vi "CCD_cinfig_to_INP.vi"(1 "Ask If Ok To Save":bool, 2 "Timing and Temperature":T4={"Exposure"=0.001, "Collection Mode"=1, "Timing Mode"=1, "Trigger Edge"=1, "Temperature"=-10.0} {"Temperature" format="%.2f"; "Trigger Edge" max=7 step=1; "Timing Mode" min=1 max=20 step=1; "Exposure" min=0.0 step=0.001 format="%.3f"}, 6 "Custom Chip":T1, 7 "ADC and Cleans":T3={"ADC Speed"=-2, "ADC Gain"=-1, "ADC Offset"=-1, "Readout Port"=-1, "Num Cleans"=1, "Num Strips per Clean"=10, "Mini Block Size"=2, "Num Min Blocks"=3, "Continous Cleans"=FALSE, "Skip Serial Reg Clean"=FALSE} {"Readout Port" min=-1 step=1; "ADC Offset" min=-1 step=1; "ADC Gain" min=-1 step=1; "ADC Speed" min=-3 step=1}, 8 "error in (no error)":errorcluster, 9 "Shutter and Logic Out":T2={"Shutter State"=2, "Open Comp Time "=0, "Close Comp Time"=0, "Logic Out Setting"=1, "Logic Out Invert"=FALSE} {"Logic Out Setting" min=1 max=14 step=1}, 10 "Camera Number":u32=1, 11 "Full File Path":string) -> (0 "error out":errorcluster)   [LabVIEW 2015]
uses:
  <vilib>/Utility/config.llb/Write Key (String).vi
  <vilib>/Utility/config.llb/Write Key (Double).vi
  <vilib>/Utility/config.llb/Write Key (U32).vi
  <vilib>/Utility/config.llb/Write Key (Boolean).vi
  <vilib>/Utility/config.llb/Write Key (I32).vi
  <vilib>/Utility/config.llb/NI_LVConfig.lvlib
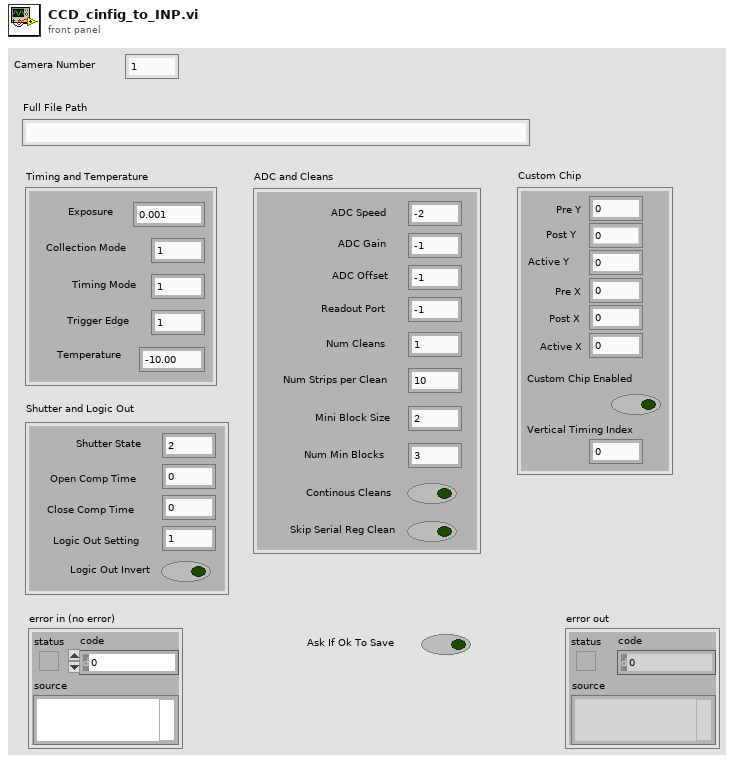
[diagram p1: front panel]
types:
  T1 = cluster{"Pre Y":u32, "Post Y":u32, "Active Y":u32, "Pre X":u32, "Post X":u32, "Active X":u32, "Custom Chip Enabled":bool, "Vertical Timing Index":u32}
  T2 = cluster{"Shutter State":u16, "Open Comp Time ":u32, "Close Comp Time":u32, "Logic Out Setting":u32, "Logic Out Invert":bool}
  T3 = cluster{"ADC Speed":i32, "ADC Gain":i32, "ADC Offset":i32, "Readout Port":i32, "Num Cleans":u32, "Num Strips per Clean":u32, "Mini Block Size":u32, "Num Min Blocks":u32, "Continous Cleans":bool, "Skip Serial Reg Clean":bool}
  T4 = cluster{"Exposure":dbl, "Collection Mode":u32, "Timing Mode":u32, "Trigger Edge":u32, "Temperature":dbl}
  T5 = typedef "NI_LVConfig.lvlib/Config Data RefNum.ctl" = refnum<k1>
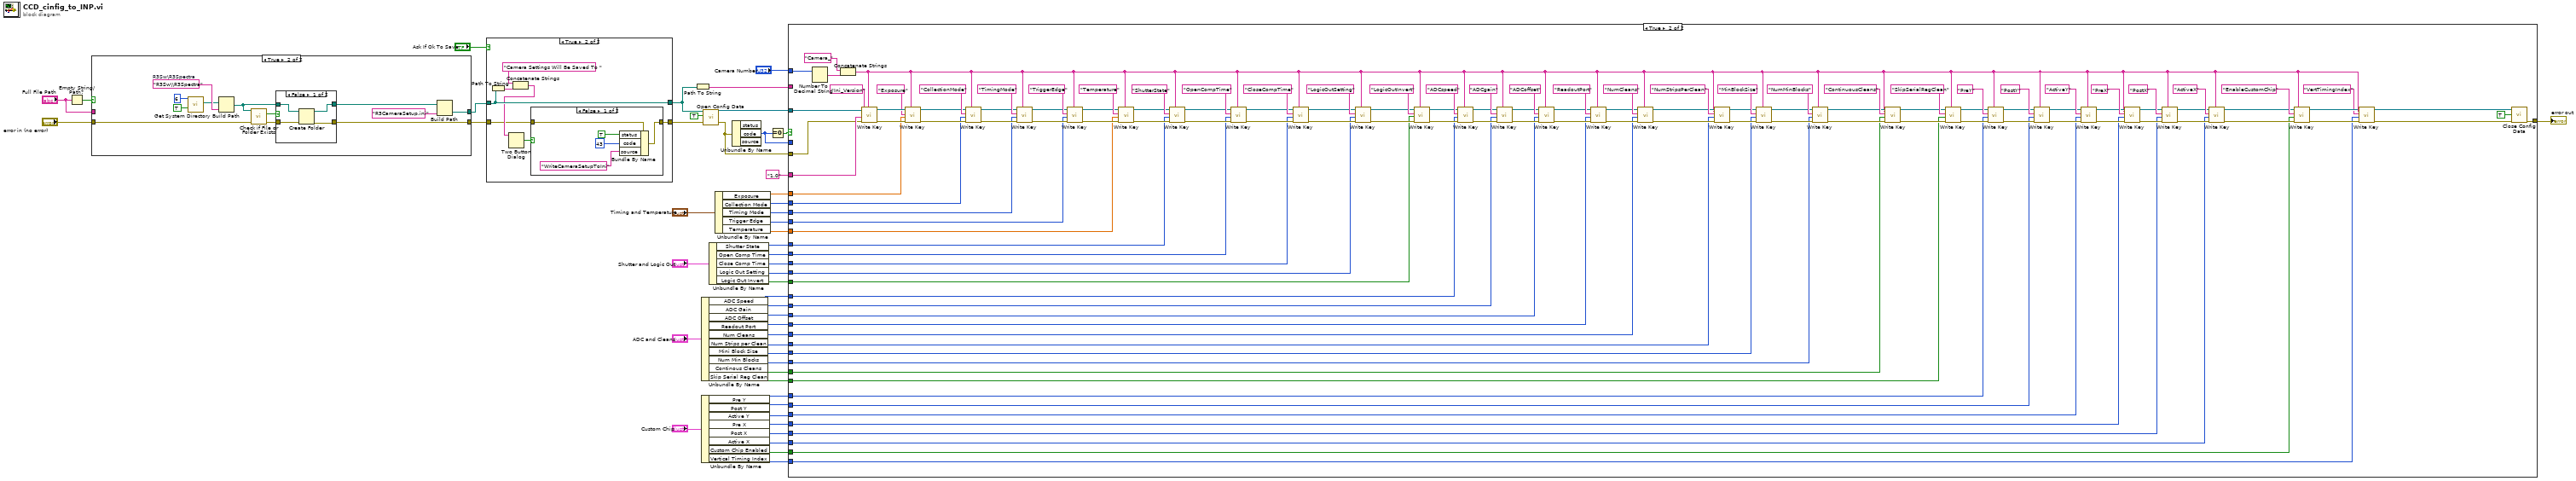
[diagram p0: block diagram]
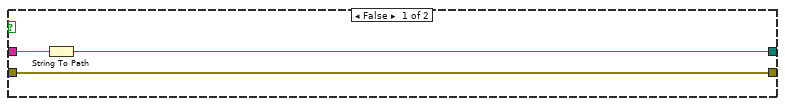
[diagram p4: hidden frame]
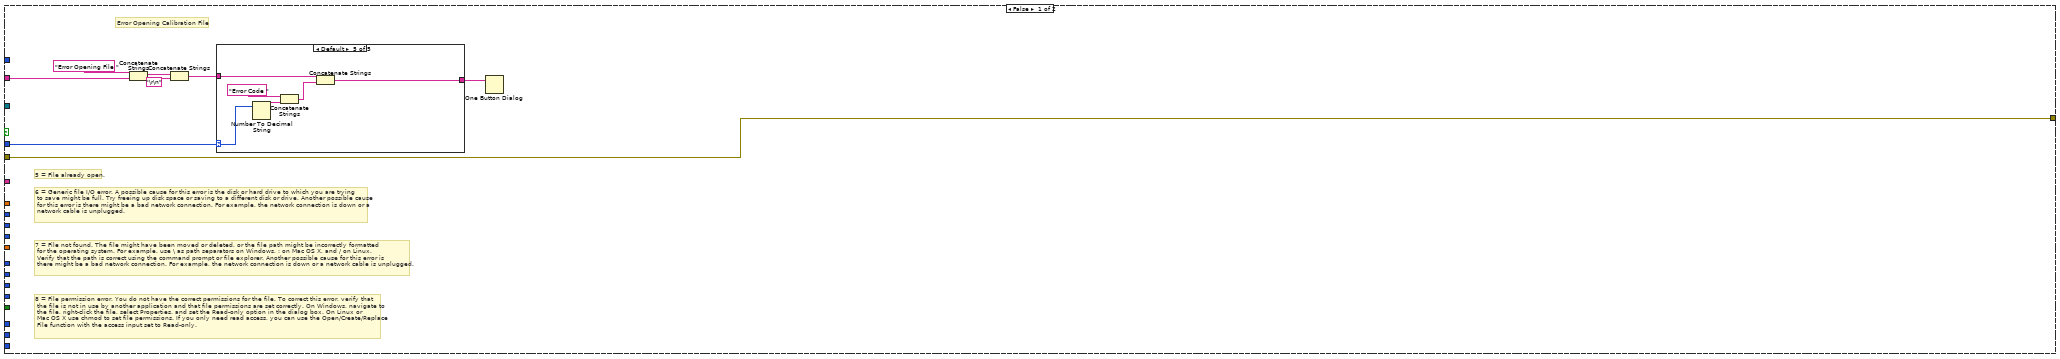
[diagram p6: hidden frame]
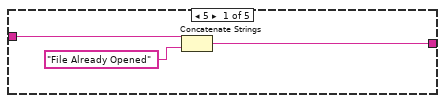
[diagram p7: hidden frame]
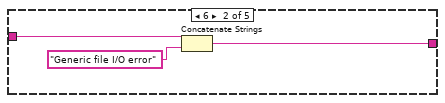
[diagram p8: hidden frame]
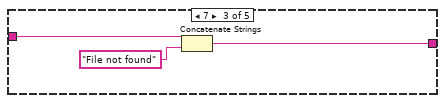
[diagram p9: hidden frame]
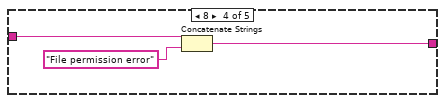
[diagram p10: hidden frame]
diagram:
  n1 = Empty String/Path?(string/path="Full File Path") -> (empty?=w39:bool)
  n2 = case shown="True" w39 {
    tunnel: [w50 w63] -> w38
    tunnel: "error in (no error)" -> [w52 w55]
    tunnel: [w52 w54] -> w36
    tunnel: "Full File Path" -> [w51 _]
    frame False {
      n3 = String To Path(string=w51) -> (path=w50:path)
    }
    frame True {
      w58 = "R3Sw\\R3Spectra"  # R3Sw\R3Spectra
      n4 = call <vilib>:"Get System Directory.vi"("create directory if not found? (F)"=TRUE, "system directory type"=6) -> ("system directory"=w57:path)  [unwired: 9 in]
      n5 = Build Path(base path=w57, name or relative path=w58) -> (appended path=w56:path)
      n6 = call <vilib>:"Check if File or Folder Exists.vi"("error in (no error)"=w55, "path"=w56) -> ("error out"=w61:errorcluster, "file or folder exists?"=w62:bool)  [unwired: 7 in, 1 out]
      n7 = case shown="False" w62 {
        tunnel: w61 -> [w67 w70]
        tunnel: [w66 w70] -> w54
        tunnel: w56 -> [w68 w69]
        tunnel: [w65 w69] -> w53
        frame False {
          n8 = Create Folder(path (use dialog)=w68, error in=w67) -> (created path=w65:path, error out=w66:errorcluster)  [unwired: 1 in, 1 out]
        }
        frame True {
        }
      }
      n9 = Build Path(base path=w53, name or relative path="R3CameraSetup.ini") -> (appended path=w63:path)
    }
  }
  n10 = case shown="True" "Ask If Ok To Save" {
    tunnel: w38 -> [w72 w79]
    tunnel: [w72 w79] -> w37
    tunnel: w36 -> [w71 w75]
    tunnel: [w71 w74] -> w35
    frame False {
    }
    frame True {
      n11 = Path To String(path=w79) -> (string=w78:string)
      n12 = Concatenate Strings("Camera Settings Will Be Saved To ", w78) -> (w76:string)
      n13 = Two Button Dialog(message=w76) -> (T button?=w73:bool)  [unwired: 2 in]
      n14 = case shown="False" w73 {
        tunnel: w75 -> [w84 w85]
        tunnel: [w83 w85] -> w74
        frame False {
          n15 = Bundle By Name(cluster=w84, "status"=TRUE, "code"=43, "source"="WriteCameraSetupToIni") -> (w83:errorcluster)
        }
        frame True {
        }
      }
    }
  }
  n16 = Path To String(path=w37) -> (string=w42:string)
  n17 = Unbundle By Name("ADC and Cleans") -> ("ADC Speed"=w19:i32, "ADC Gain"=w18:i32, "ADC Offset"=w17:i32, "Readout Port"=w16:i32, "Num Cleans"=w15:u32, "Num Strips per Clean"=w14:u32, "Mini Block Size"=w13:u32, "Num Min Blocks"=w12:u32, "Continous Cleans"=w11:bool, "Skip Serial Reg Clean"=w10:bool)
  n18 = Unbundle By Name("Custom Chip") -> ("Pre Y"=w8:u32, "Post Y"=w7:u32, "Active Y"=w6:u32, "Pre X"=w5:u32, "Post X"=w4:u32, "Active X"=w3:u32, "Custom Chip Enabled"=w2:bool, "Vertical Timing Index"=w1:u32)
  n19 = call <vilib>:"Open Config Data.vi"("error in (no error)"=w35, "create file if necessary (T)"=TRUE, "configuration file path"=w37) -> ("error out"=w46:errorcluster, "refnum"=w47:T5)  [unwired: 6 in, 1 out]
  n20 = Unbundle By Name("Shutter and Logic Out") -> ("Shutter State"=w25:u16, "Open Comp Time"=w24:u32, "Close Comp Time"=w23:u32, "Logic Out Setting"=w22:u32, "Logic Out Invert"=w21:bool)
  n21 = Unbundle By Name("Timing and Temperature") -> ("Exposure"=w31:dbl, "Collection Mode"=w30:u32, "Timing Mode"=w29:u32, "Trigger Edge"=w28:u32, "Temperature"=w27:dbl)
  n22 = Unbundle By Name(w46) -> ("code"=w45:i32)  [unwired: 2 out]
  n23 = Equal To 0?(x=w45) -> (x = 0?=w48:bool)
  n24 = case shown="True" w48 {
    tunnel: w47 -> [_ w234]
    tunnel: w46 -> [w86 w148]
    tunnel: w45 -> [w89 _]
    tunnel: w42 -> [w93 _]
    tunnel: [w86 w233] -> w44
    tunnel: "1.0" -> [_ w232]
    tunnel: "Camera Number" -> [_ w229]
    tunnel: w31 -> [_ w207]
    tunnel: w30 -> [_ w206]
    tunnel: w29 -> [_ w205]
    tunnel: w28 -> [_ w204]
    tunnel: w27 -> [_ w203]
    tunnel: w25 -> [_ w202]
    tunnel: w24 -> [_ w201]
    tunnel: w23 -> [_ w197]
    tunnel: w22 -> [_ w190]
    tunnel: w21 -> [_ w189]
    tunnel: w19 -> [_ w167]
    tunnel: w18 -> [_ w166]
    tunnel: w17 -> [_ w165]
    tunnel: w16 -> [_ w164]
    tunnel: w15 -> [_ w163]
    tunnel: w14 -> [_ w162]
    tunnel: w13 -> [_ w161]
    tunnel: w12 -> [_ w151]
    tunnel: w11 -> [_ w150]
    tunnel: w10 -> [_ w149]
    tunnel: w8 -> [_ w120]
    tunnel: w7 -> [_ w119]
    tunnel: w6 -> [_ w118]
    tunnel: w5 -> [_ w117]
    tunnel: w4 -> [_ w116]
    tunnel: w3 -> [_ w115]
    tunnel: w2 -> [_ w114]
    tunnel: w1 -> [_ w113]
    frame False {
      # "8 = File permission error. You do not have the correct permissions for the file. To correct this error, verify that\n the file is not in use by another application and that file permissions are set correctly. On Windows, navigate to\n the file, right-click the file, select Properties, and set the Read-only option in the dialog box. On Linux or\n Mac OS X use chmod to set file permissions. If you only need read access, you can use the Open/Create/Replace\n File function with the access input set to Read-only."
      # "7 = File not found. The file might have been moved or deleted, or the file path might be incorrectly formatted\n for the operating system. For example, use \\ as path separators on Windows, : on Mac OS X, and / on Linux.\n Verify that the path is correct using the command prompt or file explorer. Another possible cause for this error is\n there might be a bad network connection. For example, the network connection is down or a network cable is unplugged."
      # "6 = Generic file I/O error. A possible cause for this error is the disk or hard drive to which you are trying\n to save might be full. Try freeing up disk space or saving to a different disk or drive. Another possible cause\n for this error is there might be a bad network connection. For example, the network connection is down or a\n network cable is unplugged."
      # "5 = File already open."
      # "Error Opening Calibration File"
      n25 = Concatenate Strings("Error Opening File ", w93) -> (w90:string)
      n26 = Concatenate Strings(w90, "\r\n") -> (w88:string)
      n27 = case shown="Default" w89 {
        selector: w89 -> [_ _ _ _ w109]
        tunnel: w88 -> [w95 w98 w101 w104 w111]
        tunnel: [w94 w97 w100 w103 w110] -> w87
        frame 5 {
          n28 = Concatenate Strings(w95, "File Already Opened") -> (w94:string)
        }
        frame 6 {
          n29 = Concatenate Strings(w98, "Generic file I/O error") -> (w97:string)
        }
        frame 7 {
          n30 = Concatenate Strings(w101, "File not found") -> (w100:string)
        }
        frame 8 {
          n31 = Concatenate Strings(w104, "File permission error") -> (w103:string)
        }
        frame Default {
          n32 = Number To Decimal String(number=w109) -> (decimal integer string=w108:string)  [unwired: 1 in]
          n33 = Concatenate Strings("Error Code ", w108) -> (w106:string)
          n34 = Concatenate Strings(w111, w106) -> (w110:string)
        }
      }
      n35 = One Button Dialog(message=w87) -> ()  [unwired: 1 in, 1 out]
    }
    frame True {
      n36 = Number To Decimal String(number=w229) -> (decimal integer string=w230:string)  [unwired: 1 in]
      n37 = Concatenate Strings("Camera_", w230) -> (w126:string)
      n38 = call-poly <vilib>:"Write Key.vi"("section"=w126, "error in (no error)"=w148, "value"=w232, "key"="Ini_Version", "refnum"=w234) -> ("error out"=w227:errorcluster, "refnum out"=w228:T5)  [unwired: 4 in, 1 out]
      n39 = call-poly <vilib>:"Write Key.vi"("section"=w126, "error in (no error)"=w227, "value"=w207, "key"="Exposure", "refnum"=w228) -> ("error out"=w215:errorcluster, "refnum out"=w224:T5)  [unwired: 4 in, 1 out]
      n40 = call-poly <vilib>:"Write Key.vi"("section"=w126, "error in (no error)"=w215, "value"=w206, "key"="CollectionMode", "refnum"=w224) -> ("error out"=w214:errorcluster, "refnum out"=w222:T5)  [unwired: 4 in, 1 out]
      n41 = call-poly <vilib>:"Write Key.vi"("section"=w126, "error in (no error)"=w214, "value"=w205, "key"="TimingMode", "refnum"=w222) -> ("error out"=w213:errorcluster, "refnum out"=w220:T5)  [unwired: 4 in, 1 out]
      n42 = call-poly <vilib>:"Write Key.vi"("section"=w126, "error in (no error)"=w213, "value"=w204, "key"="TriggerEdge", "refnum"=w220) -> ("error out"=w212:errorcluster, "refnum out"=w218:T5)  [unwired: 4 in, 1 out]
      n43 = call-poly <vilib>:"Write Key.vi"("section"=w126, "error in (no error)"=w212, "value"=w203, "key"="Temperature", "refnum"=w218) -> ("error out"=w211:errorcluster, "refnum out"=w216:T5)  [unwired: 4 in, 1 out]
      n44 = call-poly <vilib>:"Write Key.vi"("section"=w126, "error in (no error)"=w211, "value"=w202, "key"="ShutterState", "refnum"=w216) -> ("error out"=w209:errorcluster, "refnum out"=w208:T5)  [unwired: 4 in, 1 out]
      n45 = call-poly <vilib>:"Write Key.vi"("section"=w126, "error in (no error)"=w209, "value"=w201, "key"="OpenCompTime", "refnum"=w208) -> ("error out"=w198:errorcluster, "refnum out"=w199:T5)  [unwired: 4 in, 1 out]
      n46 = call-poly <vilib>:"Write Key.vi"("section"=w126, "error in (no error)"=w198, "value"=w197, "key"="CloseCompTime", "refnum"=w199) -> ("error out"=w191:errorcluster, "refnum out"=w192:T5)  [unwired: 4 in, 1 out]
      n47 = call-poly <vilib>:"Write Key.vi"("section"=w126, "error in (no error)"=w191, "value"=w190, "key"="LogicOutSetting", "refnum"=w192) -> ("error out"=w193:errorcluster, "refnum out"=w194:T5)  [unwired: 4 in, 1 out]
      n48 = call-poly <vilib>:"Write Key.vi"("section"=w126, "error in (no error)"=w193, "value"=w189, "key"="LogicOutInvert", "refnum"=w194) -> ("error out"=w168:errorcluster, "refnum out"=w169:T5)  [unwired: 4 in, 1 out]
      n49 = call-poly <vilib>:"Write Key.vi"("section"=w126, "error in (no error)"=w168, "value"=w167, "key"="ADCspeed", "refnum"=w169) -> ("error out"=w183:errorcluster, "refnum out"=w186:T5)  [unwired: 4 in, 1 out]
      n50 = call-poly <vilib>:"Write Key.vi"("section"=w126, "error in (no error)"=w183, "value"=w166, "key"="ADCgain", "refnum"=w186) -> ("error out"=w182:errorcluster, "refnum out"=w184:T5)  [unwired: 4 in, 1 out]
      n51 = call-poly <vilib>:"Write Key.vi"("section"=w126, "error in (no error)"=w182, "value"=w165, "key"="ADCoffset", "refnum"=w184) -> ("error out"=w180:errorcluster, "refnum out"=w179:T5)  [unwired: 4 in, 1 out]
      n52 = call-poly <vilib>:"Write Key.vi"("section"=w126, "error in (no error)"=w180, "value"=w164, "key"="ReadoutPort", "refnum"=w179) -> ("error out"=w176:errorcluster, "refnum out"=w177:T5)  [unwired: 4 in, 1 out]
      n53 = call-poly <vilib>:"Write Key.vi"("section"=w126, "error in (no error)"=w176, "value"=w163, "key"="NumCleans", "refnum"=w177) -> ("error out"=w170:errorcluster, "refnum out"=w171:T5)  [unwired: 4 in, 1 out]
      n54 = call-poly <vilib>:"Write Key.vi"("section"=w126, "error in (no error)"=w170, "value"=w162, "key"="NumStripsPerClean", "refnum"=w171) -> ("error out"=w172:errorcluster, "refnum out"=w173:T5)  [unwired: 4 in, 1 out]
      n55 = call-poly <vilib>:"Write Key.vi"("section"=w126, "error in (no error)"=w172, "value"=w161, "key"="MinBlockSize", "refnum"=w173) -> ("error out"=w152:errorcluster, "refnum out"=w153:T5)  [unwired: 4 in, 1 out]
      n56 = call-poly <vilib>:"Write Key.vi"("section"=w126, "error in (no error)"=w152, "value"=w151, "key"="NumMinBlocks", "refnum"=w153) -> ("error out"=w154:errorcluster, "refnum out"=w155:T5)  [unwired: 4 in, 1 out]
      n57 = call-poly <vilib>:"Write Key.vi"("section"=w126, "error in (no error)"=w154, "value"=w150, "key"="ContinuousCleans", "refnum"=w155) -> ("error out"=w156:errorcluster, "refnum out"=w157:T5)  [unwired: 4 in, 1 out]
      n58 = call-poly <vilib>:"Write Key.vi"("section"=w126, "error in (no error)"=w156, "value"=w149, "key"="SkipSerialRegClean", "refnum"=w157) -> ("error out"=w128:errorcluster, "refnum out"=w127:T5)  [unwired: 4 in, 1 out]
      n59 = call-poly <vilib>:"Write Key.vi"("section"=w126, "error in (no error)"=w128, "value"=w120, "key"="PreY", "refnum"=w127) -> ("error out"=w145:errorcluster, "refnum out"=w144:T5)  [unwired: 4 in, 1 out]
      n60 = call-poly <vilib>:"Write Key.vi"("section"=w126, "error in (no error)"=w145, "value"=w119, "key"="PostY", "refnum"=w144) -> ("error out"=w141:errorcluster, "refnum out"=w142:T5)  [unwired: 4 in, 1 out]
      n61 = call-poly <vilib>:"Write Key.vi"("section"=w126, "error in (no error)"=w141, "value"=w118, "key"="ActiveY", "refnum"=w142) -> ("error out"=w135:errorcluster, "refnum out"=w136:T5)  [unwired: 4 in, 1 out]
      n62 = call-poly <vilib>:"Write Key.vi"("section"=w126, "error in (no error)"=w135, "value"=w117, "key"="PreX", "refnum"=w136) -> ("error out"=w137:errorcluster, "refnum out"=w138:T5)  [unwired: 4 in, 1 out]
      n63 = call-poly <vilib>:"Write Key.vi"("section"=w126, "error in (no error)"=w137, "value"=w116, "key"="PostX", "refnum"=w138) -> ("error out"=w129:errorcluster, "refnum out"=w130:T5)  [unwired: 4 in, 1 out]
      n64 = call-poly <vilib>:"Write Key.vi"("section"=w126, "error in (no error)"=w129, "value"=w115, "key"="ActiveX", "refnum"=w130) -> ("error out"=w131:errorcluster, "refnum out"=w132:T5)  [unwired: 4 in, 1 out]
      n65 = call-poly <vilib>:"Write Key.vi"("section"=w126, "error in (no error)"=w131, "value"=w114, "key"="EnableCustomChip", "refnum"=w132) -> ("error out"=w125:errorcluster, "refnum out"=w124:T5)  [unwired: 4 in, 1 out]
      n66 = call-poly <vilib>:"Write Key.vi"("section"=w126, "error in (no error)"=w125, "value"=w113, "key"="VertTimingIndex", "refnum"=w124) -> ("error out"=w123:errorcluster, "refnum out"=w122:T5)  [unwired: 4 in, 1 out]
      n67 = call <vilib>:"Close Config Data.vi"("error in (no error)"=w123, "write file if changed (T)"=TRUE, "refnum"=w122) -> ("error out"=w233:errorcluster)  [unwired: 7 in, 1 out]
    }
  }
  "error out" <- w44
